vi "Untitled 1.vi"() -> ()   [LabVIEW 2019]
uses:
  Communication/ABComm/Message2/Message2.lvclass
panel:
  in  "ABComm.lvlib:Message2.lvclass":refnum<class "Message2.lvclass">
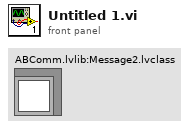
[diagram p1: front panel]
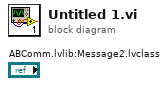
[diagram p0: block diagram]
diagram:
